vi "Hab Lifter Controller.vi"(8 "error in":errorcluster) -> ()   [LabVIEW 2018]
doc: "This VI executes continuously carrying out the current operation and responding to updates or new operations. It will often contain the timing or control code that is difficult to place directly in TeleOp. This VI generally opens all sensors and motors and isolates the rest of the robot code from knowing how the operations are carried out."
uses:
  <vilib>/Rock Robotics/WPI/Framework/Completion Status.ctl
  Hab Lifter Setpoints.ctl
  Hab Lifter Operations.ctl
  <vilib>/Rock Robotics/WPI/ThirdParty/REV Robotics/SPARK MAX/Typedef/Spark MAX Control Type.ctl
panel:
  out "Back Hab Velocity":dbl
  out "Front Hab Velocity":dbl
  in  "Interactive Values":T1
  out "Current\nCmd":string
  in  "Buttons":cluster{"Execute Cmd":bool, "Abort Cmd":bool}
  out "Command Timing":cluster{"Start Time (ms)":u32, "Iterations":i32}
  out "Status":T3
  # "Tip: It may be helpful to observe inputs and sensor values.\nYou may also want to display tuning or debugging controls."
  # "Click here to set max"
  # "Click here to set min"
  # "Interactive Command: You may fill in the settings for a command\nand schedule it with the Execute button. You can observe and abort\nany command while fine tuning the code for the controller."
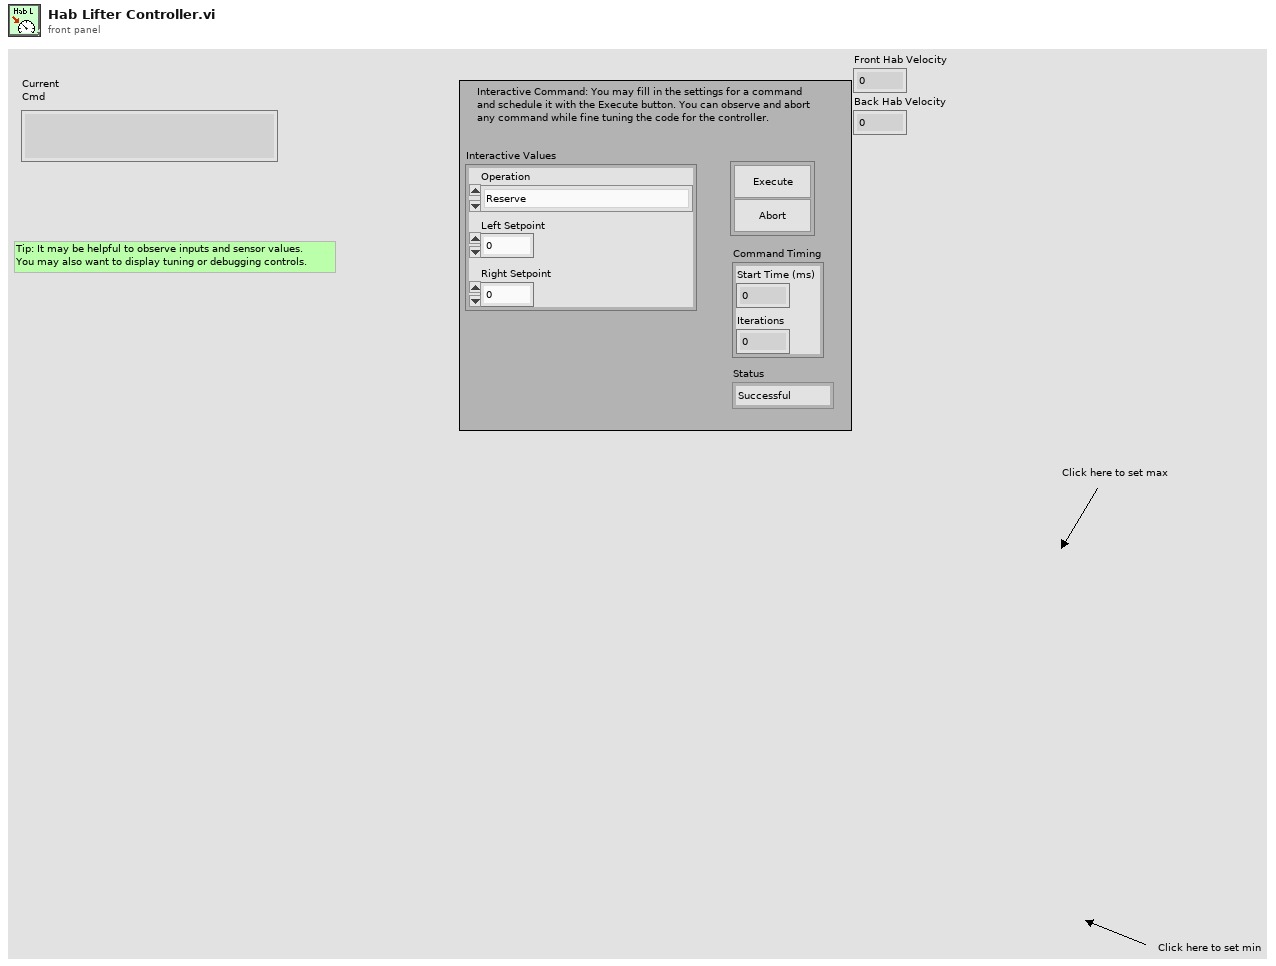
[diagram p1: front panel]
types:
  T1 = typedef "Hab Lifter Setpoints.ctl" = cluster{"Operation":T2, "Left Setpoint":dbl, "Right Setpoint":dbl}
  T2 = typedef "Hab Lifter Operations.ctl" = enum16{"Reserve", "Read Current", "Immediate"}
  T3 = typedef "Completion Status.ctl" = enum16{"Successful", "Aborted", "Incomplete"}
  T4 = cluster{"P Gain":dbl, "I Gain":dbl, "D Gain":dbl, "F Gain":dbl, "I Zone":dbl, "Min Output":dbl, "Max Output":dbl}
  T5 = typedef "WPI_MotorControlDeviceRef.ctl" = cluster{"DeviceStatus":errorcluster, "Type":T6, "PWM":cluster{"PWM Channel":T7, "DeadBand":T8}, "CAN":cluster{"Device Number":u8, "SetOutput VI Ref":variant, "GetOutput VI Ref":variant, "Enable VI Ref":variant, "Disable VI Ref":variant, "Data":variant}, "Invert":bool, "DIO PWM":cluster{"PWM \"Enable\" Channel":T7, "DIOChannel":T9, "PWM Rate":dbl}}
  T6 = typedef "WPI_MotorControlType.ctl" = enum16{"PWM", "CAN", "DIO PWM"}
  T7 = typedef "FPGA_DIOPWMChannel.ctl" = enum8{"PWM 0", "PWM 1", "PWM 2", "PWM 3", "PWM 4", "PWM 5", "PWM 6", "PWM 7", "PWM 8", "PWM 9", "PWM MXP 0", "PWM MXP 1", "PWM MXP 2", "PWM MXP 3", "PWM MXP 4", "PWM MXP 5", "PWM MXP 6", "PWM MXP 7", "PWM MXP 8", "PWM MXP 9", "Invalid"}
  T8 = typedef "WPI_PWMDeadband.ctl" = cluster{"Name":string, "maxPositivePwm":i32, "minPositivePwm":i32, "centerPwm":i32, "maxNegativePwm":i32, "minNegativePwm":i32, "angularRange":u16}
  T9 = typedef "FPGA_DIOChannel.ctl" = enum8{"DIO 0", "DIO 1", "DIO 2", "DIO 3", "DIO 4", "DIO 5", "DIO 6", "DIO 7", "DIO 8", "DIO 9", "DIO MXP 0", "DIO MXP 1", "DIO MXP 2", "DIO MXP 3", "DIO MXP 4", "DIO MXP 5", "DIO MXP 6", "DIO MXP 7", "DIO MXP 8", "DIO MXP 9", "DIO MXP 10", "DIO MXP 11", "DIO MXP 12", "DIO MXP 13", "DIO MXP 14", "DIO MXP 15", "SPI Port CS1", "SPI Port CS2", "SPI Port CS3", "SPI Port MISO", "SPI Port MOSI", "Invalid"}
  T10 = typedef "Command Status Info.ctl" = cluster{"Name":string, "Status":T3, "notifier out":T11}
  T11 = typedef "Completion Notifier.ctl" = refnum<notifier>
  T12 = cluster{"Current Command":T1, "Command Timing":cluster{"Start Time (ms)":u32, "Iterations":i32}, "Command Arguments":cluster{"Command Info":T10, "Description":string, "Default Command":T1, "queue out":refnum<queue>, "Subsystem Name":string}}
  T13 = typedef "Spark MAX Control Type.ctl" = enum16{"Percent VBus", "Voltage", "Velocity", "Position", "Smart Motion", "Current", "Smart Velocity"}
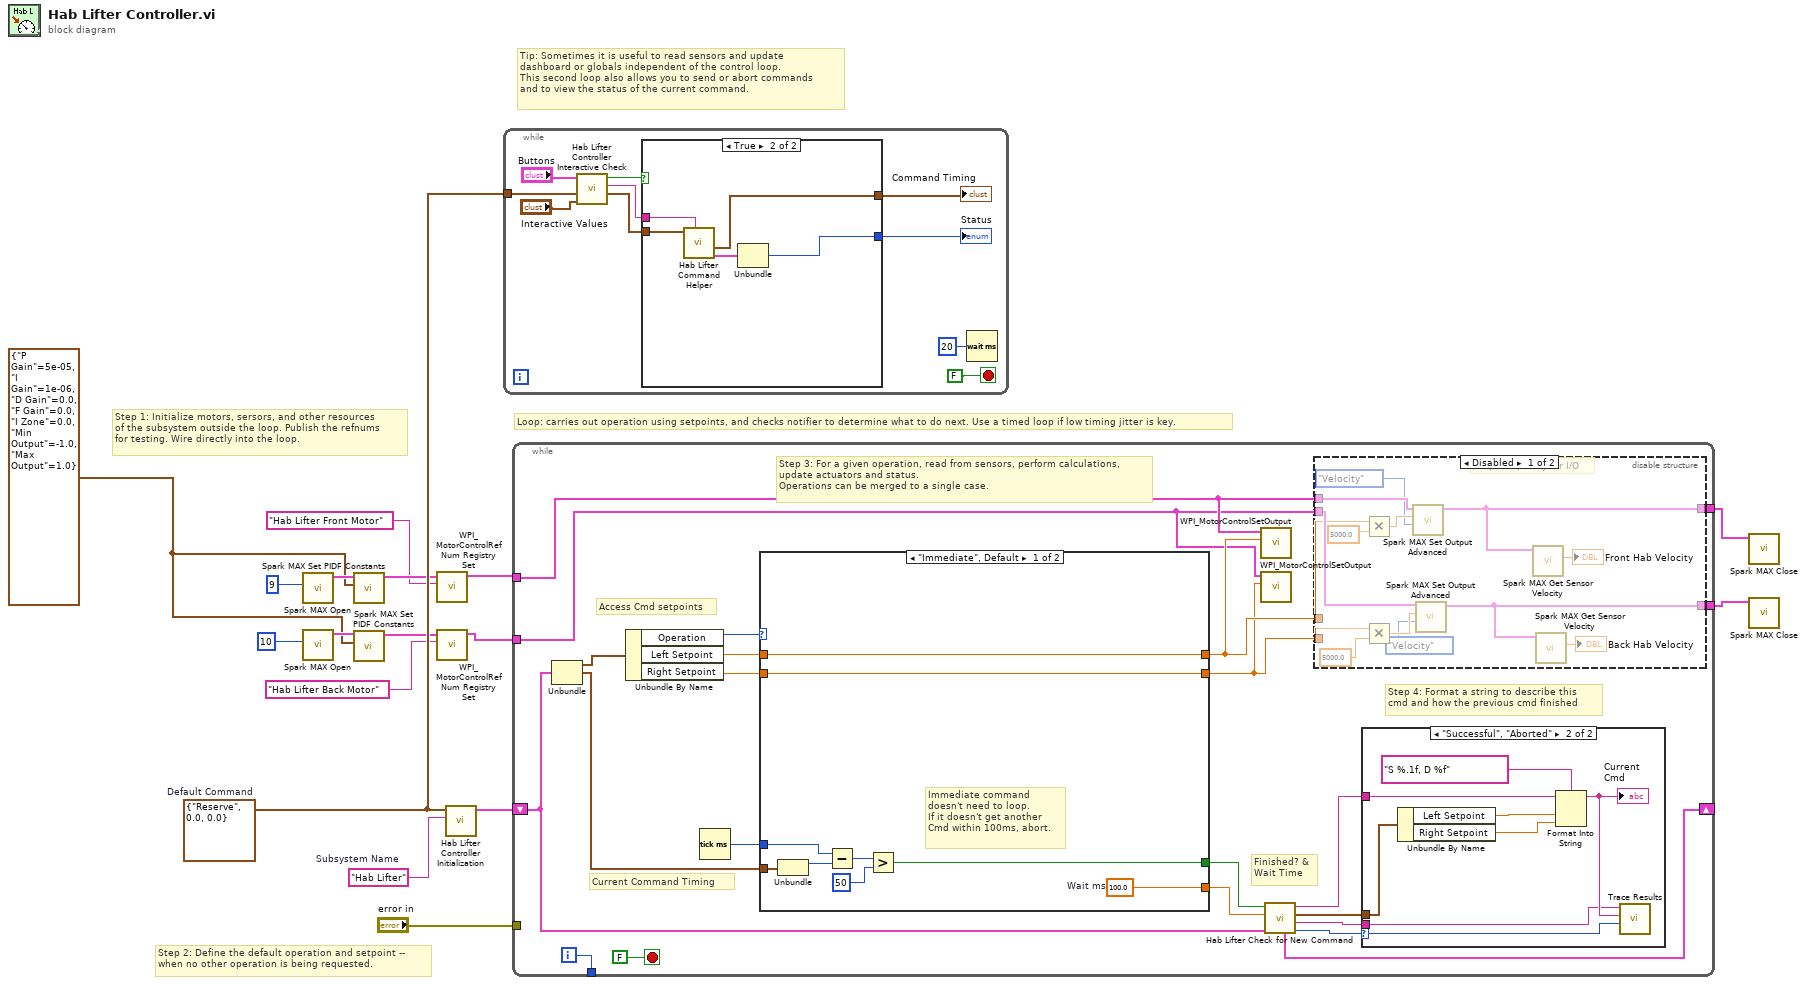
[diagram p0: block diagram]
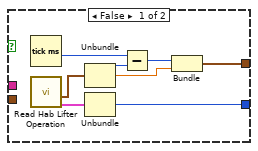
[diagram p2: hidden frame]
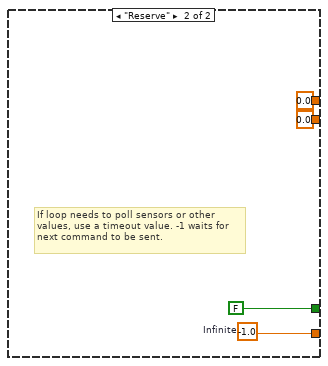
[diagram p5: hidden frame]
diagram:
  w9 = T4 {"P Gain"=5e-05, "I Gain"=1e-06, "D Gain"=0.0, "F Gain"=0.0, "I Zone"=0.0, "Min Output"=-1.0, "Max Output"=1.0} ("PID Constants")
  w14 = T1 {"Operation"=enum."Reserve", "Left Setpoint"=0.0, "Right Setpoint"=0.0}  # Default Command
  w15 = "Hab Lifter"  # Subsystem Name
  # "Tip: Sometimes it is useful to read sensors and update\ndashboard or globals independent of the control loop.\nThis second loop also allows you to send or abort commands\nand to view the status of the current command."
  # "Step 2: Define the default operation and setpoint --\nwhen no other operation is being requested."
  # "Step 1: Initialize motors, sersors, and other resources\nof the subsystem outside the loop. Publish the refnums\nfor testing. Wire directly into the loop."
  # "Loop: carries out operation using setpoints, and checks notifier to determine what to do next. Use a timed loop if low timing jitter is key."
  n1 = call <vilib>:"Spark MAX Open.vi"("Device Number"=u8 9) -> ("MotorControlDeviceRef"=w13:T5)  [unwired: 9 in, 1 out]
  n2 = call <vilib>:"Spark MAX Open.vi"("Device Number"=u8 10) -> ("MotorControlDeviceRef"=w10:T5)  [unwired: 9 in, 1 out]
  n3 = call <vilib>:"Spark MAX Set PIDF Constants.vi"("PID Constants"=w9, "MotorControlDeviceRef"=w13) -> ("MotorControlDeviceRef"=w8:T5)  [unwired: 8 in, 1 out]
  n4 = call <vilib>:"Spark MAX Set PIDF Constants.vi"("PID Constants"=w9, "MotorControlDeviceRef"=w10) -> ("MotorControlDeviceRef"=w7:T5)  [unwired: 8 in, 1 out]
  n5 = call <vilib>:"WPI_MotorControlRefNum Registry Set.vi"("refnum name"="Hab Lifter Front Motor", "MotorControlDevRef"=w8) -> ("MotorControlDevRef"=w4:T5)  [unwired: 8 in, 1 out]
  n6 = call <vilib>:"WPI_MotorControlRefNum Registry Set.vi"("refnum name"="Hab Lifter Back Motor", "MotorControlDevRef"=w7) -> ("MotorControlDevRef"=w3:T5)  [unwired: 8 in, 1 out]
  n7 = call "Hab Lifter Controller Initialization.vi"("Subsystem Name"=w15, "Default Command"=w14) -> ("Current Command"=w16:T12)  [unwired: 9 in]
  n8 = while {
    tunnel: w14 -> [w24]
    stop <- FALSE stop-if-true
    n9 = call "Hab Lifter Controller Interactive Check.vi"("Interactive Command in"="Interactive Values", "Default Command"=w24, "Buttons"="Buttons") -> ("Interactive Command out"=w21:T1, "Trace String"=w22:string, "Schedule"=w23:bool)  [unwired: 6 in]
    n10 = case shown="True" w23 {
      tunnel: [w35 w40] -> w20
      tunnel: w21 -> [_ w38]
      tunnel: [w31 w36] -> w19
      tunnel: w22 -> [_ w39]
      frame False {
        n11 = Tick Count (ms)() -> (millisecond timer value=w30:u32)
        n12 = call "Read Hab Lifter Operation.vi"() -> ("Command Info"=w28:T10, "SubSystem Data"=w29:T1)  [unwired: 9 in, 1 out]
        n13 = Unbundle(w29) -> ("Operation"=w34:T2, "Left Setpoint"=w32:dbl)  [unwired: 1 out]
        n14 = Unbundle(w28) -> ("Status"=w35:T3)  [unwired: 2 out]
        n15 = Subtract(x=w30, y=w34) -> (x-y=w33:u32)
        n16 = Bundle(w33, "Left Setpoint"=w32) -> (w31:cluster{u32, "Left Setpoint":dbl})  [unwired: 1 in]
      }
      frame True {
        n17 = call "Hab Lifter Command Helper.vi"("Description"=w39, "SubSystem Data"=w38) -> ("Command Info Out"=w37:T10, "Command Timing"=w36:cluster{"Start Time (ms)":u32, "Iterations":i32})  [unwired: 7 in, 1 out]
        n18 = Unbundle(w37) -> ("Status"=w40:T3)  [unwired: 2 out]
      }
    }
    "Status" <- w20
    "Command Timing" <- w19
    n19 = Wait (ms)(milliseconds to wait=u32 20) -> ()  [unwired: 1 out]
  }
  n20 = while {
    shift-right: [w54] -> _
    shift-left: w16 -> [w47]
    tunnel: [w61] -> _
    tunnel: "error in" -> [_]
    tunnel: w4 -> [w44]
    tunnel: w3 -> [w41]
    tunnel: [w46] -> w2
    tunnel: [w45] -> w1
    i -> [w61]
    stop <- FALSE stop-if-true
    # "Step 4: Format a string to describe this\ncmd and how the previous cmd finished"
    # "Current Command Timing"
    # "Access Cmd setpoints"
    # "Finished? &\nWait Time"
    # "Step 3: For a given operation, read from sensors, perform calculations,\nupdate actuators and status.\nOperations can be merged to a single case."
    n21 = Unbundle(w47) -> ("Current Command"=w60:T1, "Command Timing"=w56:cluster{"Start Time (ms)":u32, "Iterations":i32})  [unwired: 1 out]
    n22 = Unbundle By Name(w60) -> ("Operation"=w59:T2, "Left Setpoint"=w58:dbl, "Right Setpoint"=w55:dbl)
    n23 = Tick Count (ms)() -> (millisecond timer value=w57:u32)
    n24 = case shown="\"Immediate\", Default" w59 {
      tunnel: [w93 w97] -> w52
      tunnel: [w87 FALSE ("ignore previous (F)")] -> w53
      tunnel: w56 -> [w89 _]
      tunnel: w58 -> [w86 _]
      tunnel: w57 -> [w88 _]
      tunnel: w55 -> [w85 _]
      tunnel: [w85 0.0 ("Setpoint")] -> w42
      tunnel: [w86 0.0 ("Left Setpoint")] -> w43
      frame "Immediate", Default {
        w93 = 100.0  # Wait ms
        # "Immediate command\ndoesn't need to loop.\nIf it doesn't get another\nCmd within 100ms, abort."
        n25 = Unbundle(w89) -> ("Start Time (ms)"=w92:u32)  [unwired: 1 out]
        n26 = Subtract(x=w88, y=w92) -> (x-y=w91:u32)
        n27 = Greater?(x=w91, y=u8 50 ("Left Motor")) -> (0:w87:bool)
      }
      frame "Reserve" {
        w97 = -1.0  # Infinite
        # "If loop needs to poll sensors or other\nvalues, use a timeout value. -1 waits for\nnext command to be sent."
      }
    }
    n28 = call <vilib>:"WPI_MotorControlSetOutput.vi"("Output"=w43, "MotorControlDevRef"=w44) -> ()  [unwired: 7 in, 3 out]
    n29 = call <vilib>:"WPI_MotorControlSetOutput.vi"("Output"=w42, "MotorControlDevRef"=w41) -> ()  [unwired: 7 in, 3 out]
    n30 = call "Hab Lifter Check for New Command.vi"("Current Command"=w47, "Wait time (ms)"=w52, "Finished?"=w53) -> ("Completion"=w48:T3, "Subsystem Name"=w49:string, "Current Command"=w50:T1, "Initial Trace String"=w51:string, "NextCommand"=w54:T12)  [unwired: 4 in]
    n31 = disable-structure shown="Disabled" {
      disable-tunnel: w44 -> [w76 _]
      disable-tunnel: w41 -> [w75 _]
      disable-tunnel: w43 -> [w74 _]
      disable-tunnel: w42 -> [w73 _]
      disable-tunnel: [w66 _] -> w46
      disable-tunnel: [w65 _] -> w45
      frame Disabled {
        # "Step 5: Upate your I/O"
        n32 = Multiply(x=w74, y=5000.0) -> (x*y=w71:dbl)
        n33 = Multiply(x=w73, y=5000.0) -> (x*y=w68:dbl)
        n34 = call <vilib>:"Spark MAX Set Output Advanced.vi"("Control Mode"=Spark_MAX_Control_Type."Velocity", "Setpoint"=w71, "MotorControlDevRef"=w76) -> ("MotorControlDevRef"=w66:T5)  [unwired: 7 in, 1 out]
        n35 = call <vilib>:"Spark MAX Set Output Advanced.vi"("Control Mode"=Spark_MAX_Control_Type."Velocity", "Setpoint"=w68, "MotorControlDevRef"=w75) -> ("MotorControlDevRef"=w65:T5)  [unwired: 7 in, 1 out]
        n36 = call <vilib>:"Spark MAX Get Sensor Velocity.vi"("MotorControlDevRef in"=w66) -> ("Sensor Velocity"=→"Front Hab Velocity":dbl)  [unwired: 7 in, 3 out]
        n37 = call <vilib>:"Spark MAX Get Sensor Velocity.vi"("MotorControlDevRef in"=w65) -> ("Sensor Velocity"=→"Back Hab Velocity":dbl)  [unwired: 7 in, 3 out]
      }
      frame Enabled {
      }
    }
    n38 = case shown="\"Successful\", \"Aborted\"" w48 {
      selector: w48 -> [_ w84]
      tunnel: w51 -> [_ w80]
      tunnel: w50 -> [_ w81]
      tunnel: w49 -> [_ w77]
      frame "Incomplete", Default {
        # "Continuing current command"
      }
      frame "Successful", "Aborted" {
        # "Report and setup for next command"
        n39 = Unbundle By Name(w81) -> ("Left Setpoint"=w83:dbl, "Right Setpoint"=w78:dbl)
        n40 = Format Into String(format string="S %.1f, D %f", initial string=w80, w83, w78) -> (resulting string=w79:string)  [unwired: 1 in, 1 out]
        "Current\nCmd" <- w79
        n41 = call <vilib>:"Trace Results.vi"("Status of previous command"=w84, "Description"=w79, "Subsystem"=w77) -> ()  [unwired: 9 in]
      }
    }
  }
  n42 = call <vilib>:"Spark MAX Close.vi"("MotorControlDeviceRef"=w2) -> ()  [unwired: 10 in, 1 out]
  n43 = call <vilib>:"Spark MAX Close.vi"("MotorControlDeviceRef"=w1) -> ()  [unwired: 10 in, 1 out]
